vi "sub_enqueue commands.vi"(10 "commands":string[](array[string]), 11 "Queue in":refnum<queue>) -> ()   [LabVIEW 2018]
panel:
  in  "enqueue at opposite end ?":bool
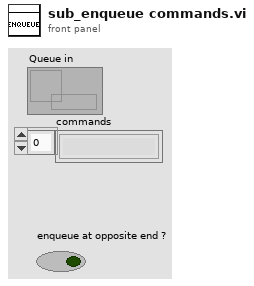
[diagram p1: front panel]
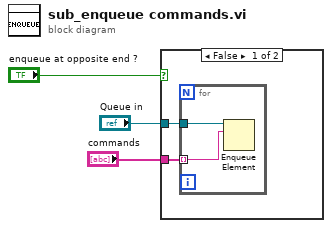
[diagram p0: block diagram]
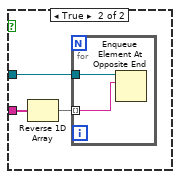
[diagram p2: hidden frame]
diagram:
  n1 = case shown="False" "enqueue at opposite end ?" {
    tunnel: "commands" -> [w5 w10]
    tunnel: "Queue in" -> [w4 w9]
    frame False {
      n2 = for {
        tunnel: w4 -> [w7]
        tunnel: w5 -> [w6] mode=indexing
        n3 = Enqueue Element(queue=w7, element=w6) -> ()  [unwired: 2 in, 3 out]
      }
    }
    frame True {
      n4 = Reverse 1D Array(array=w10) -> (reversed array=w8:string[])
      n5 = for {
        tunnel: w9 -> [w12]
        tunnel: w8 -> [w11] mode=indexing
        n6 = Enqueue Element At Opposite End(queue=w12, element=w11) -> ()  [unwired: 2 in, 3 out]
      }
    }
  }
